vi "Write Ch.vi"(8 "error in":errorcluster, 9 "Channel":i32, 10 "Producer Ch":T1, 11 "Cycler Cluster - 24 Channel.lvclass":refnum<class "Cycler Cluster - 6 Channel.lvclass">) -> (0 "error out":errorcluster, 3 "output cluster":refnum<class "Cycler Cluster - 6 Channel.lvclass">)   [LabVIEW 2023, in "Cycler Cluster - 6 Channel.lvclass"]
uses:
  Cycler Cluster - 6 Channel.lvclass
  Cycler Cluster - 6 Channel.lvclass/Cycler Cluster - 6 Channel.ctl
  f4d7046b-01d5-476e-969f-edff788d7dd0.vi
  09ba8855-a333-4b05-9fa0-f00f0d112976.vi
  f692a3ce-3a89-48d1-896d-de4404ed547f.vi
  300b3033-2680-412c-ab22-c723e8d8dc08.vi
  7cf0eb00-689e-4e52-8b4d-642b65507f98.vi
  b87ff49e-8005-4a7c-bf49-406770351efc.vi
  f4d7046b-01d5-476e-969f-edff788d7dd0.vi/4bc1c15b-36ab-481f-b8dd-c64075ce723a.vi
  f4d7046b-01d5-476e-969f-edff788d7dd0.vi/d83cb72b-7713-41fc-a3d1-682de79cf574.vi
  09ba8855-a333-4b05-9fa0-f00f0d112976.vi/4bc1c15b-36ab-481f-b8dd-c64075ce723a.vi
  09ba8855-a333-4b05-9fa0-f00f0d112976.vi/d83cb72b-7713-41fc-a3d1-682de79cf574.vi
  f692a3ce-3a89-48d1-896d-de4404ed547f.vi/4bc1c15b-36ab-481f-b8dd-c64075ce723a.vi
  f692a3ce-3a89-48d1-896d-de4404ed547f.vi/d83cb72b-7713-41fc-a3d1-682de79cf574.vi
  300b3033-2680-412c-ab22-c723e8d8dc08.vi/4bc1c15b-36ab-481f-b8dd-c64075ce723a.vi
  300b3033-2680-412c-ab22-c723e8d8dc08.vi/d83cb72b-7713-41fc-a3d1-682de79cf574.vi
  7cf0eb00-689e-4e52-8b4d-642b65507f98.vi/4bc1c15b-36ab-481f-b8dd-c64075ce723a.vi
  7cf0eb00-689e-4e52-8b4d-642b65507f98.vi/d83cb72b-7713-41fc-a3d1-682de79cf574.vi
  b87ff49e-8005-4a7c-bf49-406770351efc.vi/4bc1c15b-36ab-481f-b8dd-c64075ce723a.vi
  b87ff49e-8005-4a7c-bf49-406770351efc.vi/d83cb72b-7713-41fc-a3d1-682de79cf574.vi
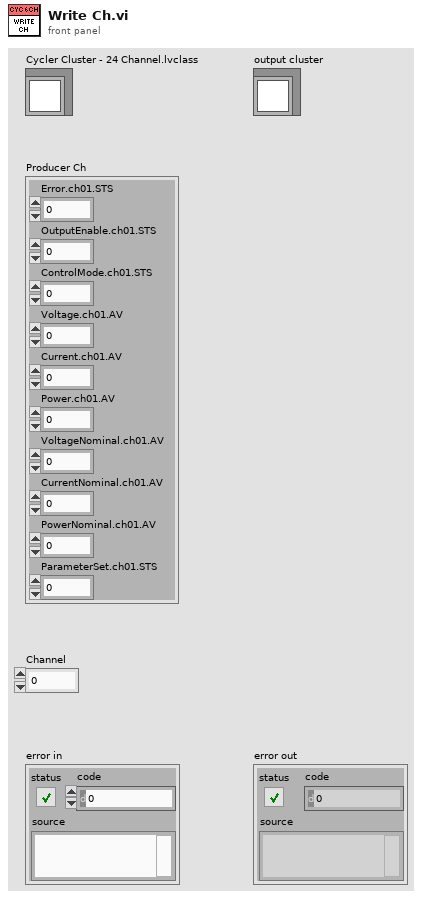
[diagram p1: front panel]
types:
  T1 = cluster{"Error.ch01.STS":i32, "OutputEnable.ch01.STS":i32, "ControlMode.ch01.STS":u16, "Voltage.ch01.AV":dbl, "Current.ch01.AV":dbl, "Power.ch01.AV":dbl, "VoltageNominal.ch01.AV":dbl, "CurrentNominal.ch01.AV":dbl, "PowerNominal.ch01.AV":dbl, "ParameterSet.ch01.STS":i32}
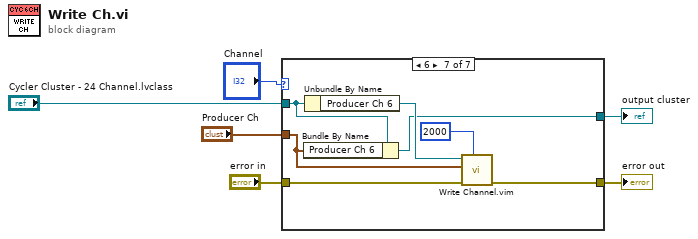
[diagram p0: block diagram]
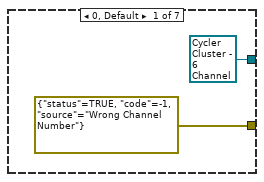
[diagram p2: hidden frame]
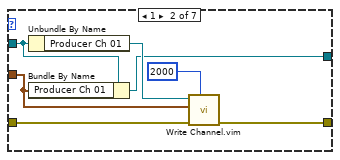
[diagram p3: hidden frame]
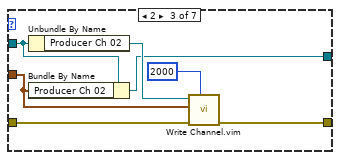
[diagram p4: hidden frame]
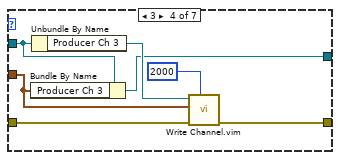
[diagram p5: hidden frame]
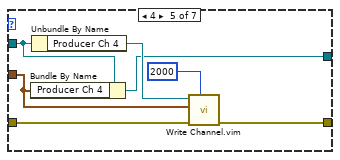
[diagram p6: hidden frame]
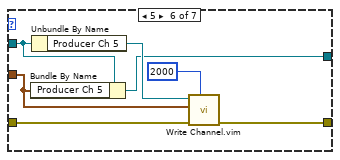
[diagram p7: hidden frame]
diagram:
  n1 = case shown="6" "Channel" {
    tunnel: "Producer Ch" -> [_ w12 w19 w26 w33 w40 w47]
    tunnel: "Cycler Cluster - 24 Channel.lvclass" -> [_ w13 w20 w27 w34 w41 w48]
    tunnel: [errorcluster {"status"=TRUE, "code"=-1, "source"="Wrong Channel Number"} ("error out") w11 w18 w25 w32 w39 w46] -> w3
    tunnel: "error in" -> [_ w10 w17 w24 w31 w38 w45]
    tunnel: [refnum<class "Cycler Cluster - 6 Channel.lvclass"> refnum ("Cycler Cluster - 24 Channel.lvclass") w9 w16 w23 w30 w37 w44] -> w1
    frame 0, Default {
    }
    frame 1 {
      n2 = Unbundle By Name(w13) -> ("Producer Ch 01"=w15:refnum<k21>)
      n3 = Bundle By Name(cluster=w13, "Producer Ch 01"=w12) -> (w9:refnum<class "Cycler Cluster - 6 Channel.lvclass">)
      n4 = call "Write Channel.vim"("Timeout (ms)"=2000, "error in"=w10, "Data in"=w12, "ADAS HIL Channel in"=w15) -> ("error out"=w11:errorcluster)  [unwired: 5 in, 2 out]
    }
    frame 2 {
      n5 = Unbundle By Name(w20) -> ("Producer Ch 02"=w22:refnum<k21>)
      n6 = Bundle By Name(cluster=w20, "Producer Ch 02"=w19) -> (w16:refnum<class "Cycler Cluster - 6 Channel.lvclass">)
      n7 = call "Write Channel.vim"("Timeout (ms)"=2000, "error in"=w17, "Data in"=w19, "ADAS HIL Channel in"=w22) -> ("error out"=w18:errorcluster)  [unwired: 5 in, 2 out]
    }
    frame 3 {
      n8 = Bundle By Name(cluster=w27, "Producer Ch 3"=w26) -> (w23:refnum<class "Cycler Cluster - 6 Channel.lvclass">)
      n9 = Unbundle By Name(w27) -> ("Producer Ch 3"=w29:refnum<k21>)
      n10 = call "Write Channel.vim"("Timeout (ms)"=2000, "error in"=w24, "Data in"=w26, "ADAS HIL Channel in"=w29) -> ("error out"=w25:errorcluster)  [unwired: 5 in, 2 out]
    }
    frame 4 {
      n11 = Bundle By Name(cluster=w34, "Producer Ch 4"=w33) -> (w30:refnum<class "Cycler Cluster - 6 Channel.lvclass">)
      n12 = Unbundle By Name(w34) -> ("Producer Ch 4"=w36:refnum<k21>)
      n13 = call "Write Channel.vim"("Timeout (ms)"=2000, "error in"=w31, "Data in"=w33, "ADAS HIL Channel in"=w36) -> ("error out"=w32:errorcluster)  [unwired: 5 in, 2 out]
    }
    frame 5 {
      n14 = Bundle By Name(cluster=w41, "Producer Ch 5"=w40) -> (w37:refnum<class "Cycler Cluster - 6 Channel.lvclass">)
      n15 = Unbundle By Name(w41) -> ("Producer Ch 5"=w43:refnum<k21>)
      n16 = call "Write Channel.vim"("Timeout (ms)"=2000, "error in"=w38, "Data in"=w40, "ADAS HIL Channel in"=w43) -> ("error out"=w39:errorcluster)  [unwired: 5 in, 2 out]
    }
    frame 6 {
      n17 = Bundle By Name(cluster=w48, "Producer Ch 6"=w47) -> (w44:refnum<class "Cycler Cluster - 6 Channel.lvclass">)
      n18 = Unbundle By Name(w48) -> ("Producer Ch 6"=w50:refnum<k21>)
      n19 = call "Write Channel.vim"("Timeout (ms)"=2000, "error in"=w45, "Data in"=w47, "ADAS HIL Channel in"=w50) -> ("error out"=w46:errorcluster)  [unwired: 5 in, 2 out]
    }
  }
  "error out" <- w3
  "output cluster" <- w1
